vi "InitParams.vi"(10 "Cluster":T1={"API Root"="", "verify server"=FALSE, "Version (no version)"="", "Port (protocol specific)"=0, "Base URL"="", "Auth type"=enum."Token", "Auth string"="", "timeout (10000)"=10000}, 11 "RESTLoaderConstant in":refnum<class "RESTLoaderConstant.lvclass">) -> (3 "RESTLoaderConstant out":refnum<class "RESTLoaderConstant.lvclass">)   [LabVIEW 2019, in "ByteREST.lvlib" / "RESTLoaderConstant.lvclass"]
uses:
  RESTLoaderConstant.lvclass
  LoaderBase/ServerParams.ctl
  ByteRESTClass/ByteRESTBase/Auth/Authentication_type.ctl
  RESTLoaderConstant.lvclass/RESTLoaderConstant.ctl
  ByteRESTClass/ByteRESTBase/RESTBase.lvclass
  LoaderBase/RESTLoaderBase.lvclass
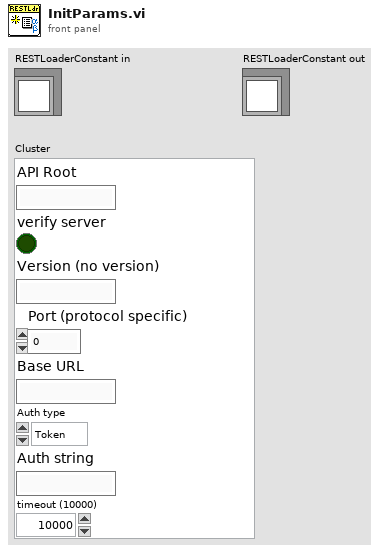
[diagram p1: front panel]
types:
  T1 = typedef "ByteREST.lvlib/RESTLoaderBase.lvclass/ServerParams.ctl" = cluster{"API Root":string, "verify server":bool, "Version (no version)":string, "Port (protocol specific)":u16, "Base URL":string, "Auth type":T2, "Auth string":string, "timeout (10000)":i32}
  T2 = typedef "ByteREST.lvlib/RESTBase.lvclass/Authentication_type.ctl" = enum16{"Token"}
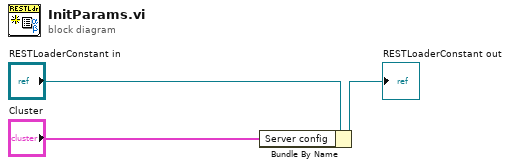
[diagram p0: block diagram]
diagram:
  n1 = Bundle By Name(cluster="RESTLoaderConstant in", "Server config"="Cluster") -> (→"RESTLoaderConstant out":refnum<class "RESTLoaderConstant.lvclass">)
